vi "BadEncoder.vi"(10 "SporaticValue":dbl) -> (2 "FixedValue":dbl)   [LabVIEW 2020]
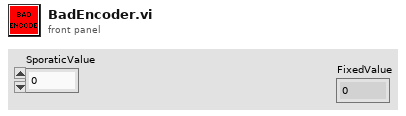
[diagram p1: front panel]
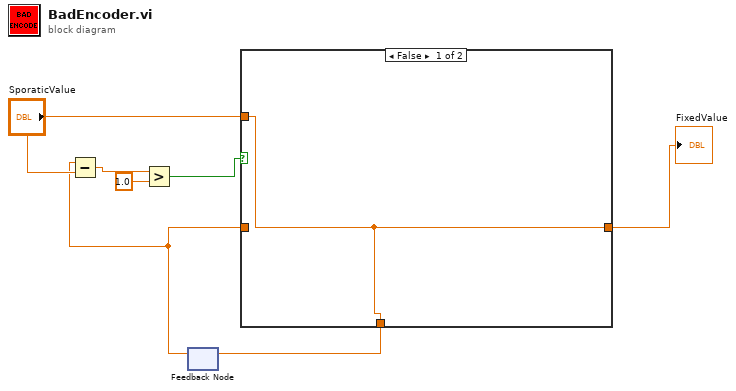
[diagram p0: block diagram]
diagram:
  n1 = feedback #1() -> (w1:dbl)  [unwired: 1 in]
  n2 = Subtract(x=w1, y="SporaticValue") -> (x-y=w5:dbl)
  n3 = Greater?(x=w5, y=1.0) -> (0:w3:bool)
  n4 = case shown="False" w3 {
    tunnel: [w8 w9] -> w7
    tunnel: w1 -> [_ w9]
    tunnel: [w8 w9] -> w6
    tunnel: "SporaticValue" -> [w8 _]
    frame False {
    }
    frame True {
    }
  }
  "FixedValue" <- w7
  n5 = feedback-in #1(w6) -> ()
